vi "Analog Input Voltages.vi"(8 "error in (no error)":errorcluster, 10 "Analog Input Voltages":waveform(dbl)[](array[waveform]), 11 "FC2901 in":refnum<class "FC2901.lvclass">) -> (0 "error out":errorcluster, 3 "FC2901 out":refnum<class "FC2901.lvclass">)   [LabVIEW 2021, in "FC2901.lvclass"]
uses:
  FC2901.lvclass
  FC2901.lvclass/FC2901.ctl
  <vilib>/Analysis/NI_AALPro.lvlib
  <vilib>/ActorFramework/Actor/Actor.lvclass
  Mass Flow Controllers/Mass Flow Controllers Messages/MFC Flow Msg/MFC Flow Msg.lvclass
  C:/Program Files/National Instruments/LabVIEW 2021/vi.lib/MGI/Panel Manager/Panel Actor/Panel Actor/Panel Actor.lvclass
  C:/Program Files/National Instruments/LabVIEW 2021/vi.lib/ActorFramework/Actor/Actor.lvclass
  C:/git/Mass-Flow-Controllers/Source/FC2901/FC2901/FC2901.lvclass
  C:/Program Files/National Instruments/LabVIEW 2021/vi.lib/NathanCo/Analog Tasks/Analog Input/Analog Input Interface Messages/Analog Input Interface Messages/Analog Input Interface Messages.lvclass
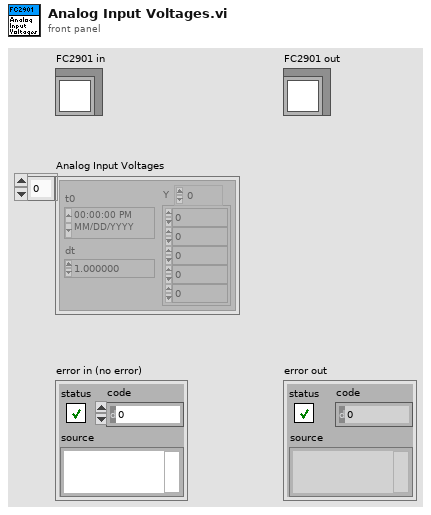
[diagram p1: front panel]
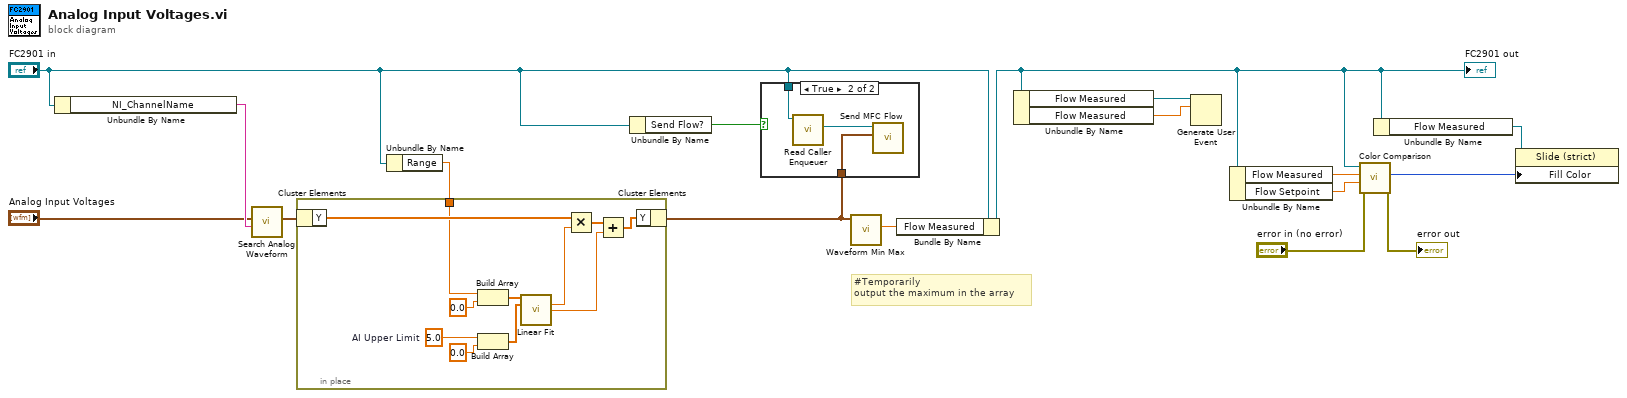
[diagram p0: block diagram]
diagram:
  # "#Temporarily\noutput the maximum in the array"
  n1 = Unbundle By Name("FC2901 in") -> ("NI_ChannelName"=w7:string)
  n2 = call <vilib>:"Search Analog Waveform.vi"("NI_ChannelName"=w7, "Waveforms"="Analog Input Voltages") -> ("Waveform"=w6:waveform(dbl))  [unwired: 8 in, 1 out]
  n3 = Unbundle By Name("FC2901 in") -> ("Range"=w8:dbl)
  n4 = in-place {
    in-place-border: w8 -> [w18]
    w26 = 5.0  # AI Upper Limit
    n5 = in-place-cluster #1(w6) -> ("Y"=w23:dbl[])
    n6 = Build Array(w18, 0.0 ("element")) -> (w27:dbl[])
    n7 = Build Array(w26, 0.0 ("minimum (EGU)")) -> (w28:dbl[])
    n8 = call <vilib>:"Linear Fit.vi"("Y"=w27, "X"=w28) -> ("slope"=w22:dbl, "intercept"=w20:dbl)  [unwired: 9 in, 3 out]
    n9 = Multiply(x=w23, y=w22) -> (x*y=w21:dbl[])
    n10 = Add(x=w21, y=w20) -> (x+y=w19:dbl[])
    n11 = in-place-cluster #1("Y"=w19) -> (w10:waveform(dbl))
  }
  n12 = Unbundle By Name("FC2901 in") -> ("Send Flow?"=w9:bool)
  n13 = case shown="True" w9 {
    tunnel: "FC2901 in" -> [_ w31]
    tunnel: w10 -> [_ w29]
    frame False {
    }
    frame True {
      n14 = call <vilib>:"Read Caller Enqueuer.vi"("Actor"=w31) -> ("Caller Enqueuer"=w30:refnum<class "Message Enqueuer.lvclass">)  [unwired: 10 in]
      n15 = call "Send MFC Flow.vi"("MFC Flow"=w29, "Message Enqueuer"=w30) -> ()  [unwired: 8 in, 2 out]
    }
  }
  n16 = call <vilib>:"Waveform Min Max.vi"("waveform in"=w10) -> ("Y max"=w11:dbl)  [unwired: 5 in, 5 out]
  n17 = Bundle By Name(cluster="FC2901 in", "Flow Measured"=w11) -> (w4:refnum<class "FC2901.lvclass">)
  "FC2901 out" <- w4
  n18 = Unbundle By Name(w4) -> ("Flow Measured"=w16:refnum<user-event>, "Flow Measured"=w15:dbl)
  n19 = Generate User Event(user event=w16, event data cluster=w15) -> ()  [unwired: 2 in, 2 out]
  n20 = Unbundle By Name(w4) -> ("Flow Measured"=w13:dbl, "Flow Setpoint"=w12:dbl)
  n21 = call "Color Comparison.vi"("error in (no error)"="error in (no error)", "Setpoint"=w12, "Level"=w13, "FC2901 in"=w4) -> ("error out"=→"error out":errorcluster, "Color"=w14:u32)  [unwired: 6 in]
  n22 = Unbundle By Name(w4) -> ("Flow Measured"=w17:refnum<vi>)
  n23 = property class="Slide (strict)"(reference=w17, "Fill Color"=w14) -> ()  [unwired: 1 in, 2 out]
